vi "PH_VacuumControl.PC Set Trend Channel.vi"(0 "i ref in":refnum<vi>, 2 "Trend Channel":u16, 5 "error IO":errorcluster) -> (14 "i ref out":refnum<vi>, 19 "error out":errorcluster)   [LabVIEW 2014, in "PH_VacuumControl.lvlib"]
doc: "This VI sets the Trend Channel to own attributes and the related GUI element."
uses:
  PH_VacuumControl.lvlib
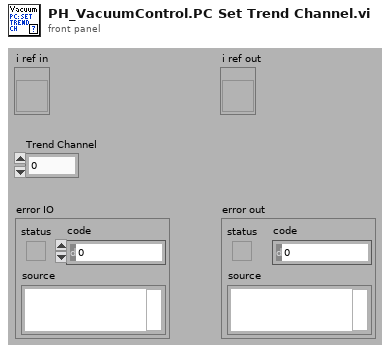
[diagram p1: front panel]
types:
  T1 = typedef "PH_VacuumControl.lvlib/PH_VacuumControl.i attribute.ctl" = cluster{"GUI Refs":cluster{"Exit":refnum<vi>, "Set Unit":refnum<vi>, "Device found":refnum<vi>, "Busy":refnum<vi>, "State":refnum<vi>, "Delete":refnum<vi>, "Channels":refnum<vi>, "Channel Name":refnum<vi>, "Trend":refnum<vi>, "Logarithmic":refnum<vi>, "Limit reached":refnum<vi>, "Channel Name 1 MT":refnum<vi>, "Channel Name 2 MT":refnum<vi>, "Trend MT":refnum<vi>, "Logarithmic MT":refnum<vi>, "Limit reached MT":refnum<vi>}, "Device found":bool, "Busy":bool, "Selected Unit":i32, "Channels [mbar]":T2, "Channel Names":cluster{"Channel 1":string, "Channel 2":string, "Channel 3":string, "Channel 4":string, "Channel 5":string, "Channel 6":string}, "Status":T3, "AGCxxx VISA Cluster":T4, "Instr Firmware Revision":string, "Service IDs Pressure":cluster{"Channel 1":i32, "Channel 2":i32, "Channel 3":i32, "Channel 4":i32, "Channel 5":i32, "Channel 6":i32}, "Service IDs Limits":cluster{"Channel 1":i32, "Channel 2":i32, "Channel 3":i32, "Channel 4":i32, "Channel 5":i32, "Channel 6":i32}, "Trend":cluster{"Start Point":timestamp, "Pressures [mbar] Channel 1":dbl[], "Pressures [mbar] Channel 2":dbl[], "Pressures [mbar] Channel 3":dbl[], "Pressures [mbar] Channel 4":dbl[], "Pressures [mbar] Channel 5":dbl[], "Pressures [mbar] Channel 6":dbl[], "Timebase [s]":i32[], "Trend Channel":u16, "Start Fit":dbl, "Trend Channel 1 MT":u16, "Trend Channel 2 MT":u16, "Start or continue Fit MT":dbl, "Continue or start Fit MT":dbl, "Datasets strored":i32, "Dataarray Size":i32}, "Running":bool}
  T2 = typedef "PH_VacuumControl.lvlib/PH_VacuumControl.Channels.ctl" = cluster{"Channel 1":dbl, "Channel 2":dbl, "Channel 3":dbl, "Channel 4":dbl, "Channel 5":dbl, "Channel 6":dbl, "Name Channel 1":string, "Name Channel 2":string, "Name Channel 3":string, "Name Channel 4":string, "Name Channel 5":string, "Name Channel 6":string, "Upper Limit":dbl, "Upper Limit 2":dbl, "Upper Limit 3":dbl, "Upper Limit 4":dbl, "Upper Limit 5":dbl, "Upper Limit 6":dbl}
  T3 = typedef "PH_StatusHandler.lvlib/PH_StatusHandler.Status.ctl" = i16
  T4 = typedef "AGCxxx - Driver.lvlib/AGCxxx VISA Control.ctl" = cluster{"VISA resource name":refnum<visa-resource-name>, "VISA Timeout Value (1000 ms)":u32, "Lock Timeout (1000 ms)":u32, "MAX Channel (6)":i32}
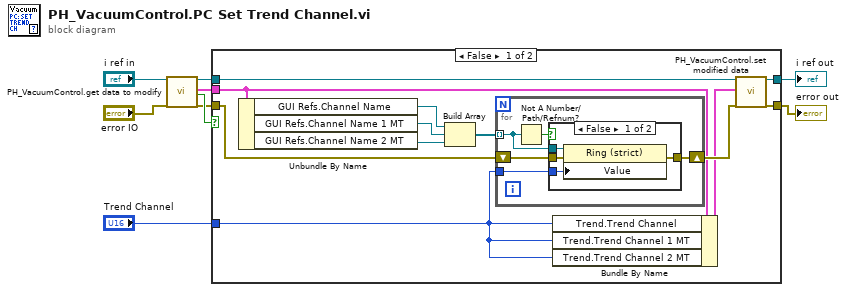
[diagram p0: block diagram]
diagram:
  n1 = call "PH_VacuumControl.get data to modify.vi"("i ref in"="i ref in", "error in (no error)"="error IO") -> ("i ref out"=w7:refnum<vi>, "i attribute"=w3:T1, "timed out"=w6:bool, "error out"=w4:errorcluster)  [unwired: 14 in]
  n2 = case shown="False" w6 {
    tunnel: w3 -> [w16 _]
    tunnel: w4 -> [w20 w32]
    tunnel: [w19 w32] -> w5
    tunnel: w7 -> [w18 w33]
    tunnel: [w17 w33] -> w8
    tunnel: "Trend Channel" -> [w14 _]
    frame False {
      n3 = Unbundle By Name(w16) -> ("GUI Refs.Channel Name"=w13:refnum<vi>, "GUI Refs.Channel Name 1 MT"=w11:refnum<vi>, "GUI Refs.Channel Name 2 MT"=w10:refnum<vi>)
      n4 = Build Array(w13, w11, w10) -> (w12:refnum<vi>[])
      n5 = for {
        tunnel: w14 -> [w23]
        tunnel: w12 -> [w22] mode=indexing
        shift-right: [w26] -> w21
        shift-left: w20 -> [w25]
        n6 = Not A Number/Path/Refnum?(number/path/refnum=w22) -> (NaN/Path/Refnum?=w24:bool)
        n7 = case shown="False" w24 {
          tunnel: [w30 w31] -> w26
          tunnel: w25 -> [w29 w31]
          tunnel: w22 -> [w28 _]
          tunnel: w23 -> [w27 _]
          frame False {
            n8 = property class="Ring (strict)"(reference=w28, error in=w29, "Value"=w27) -> (error out=w30:errorcluster)  [unwired: 1 out]
          }
          frame True {
          }
        }
      }
      n9 = Bundle By Name(cluster=w16, "Trend.Trend Channel"=w14, "Trend.Trend Channel 1 MT"=w14, "Trend.Trend Channel 2 MT"=w14) -> (w15:T1)
      n10 = call "PH_VacuumControl.set modified data.vi"("i ref in"=w18, "i attribute"=w15, "error in (no error)"=w21) -> ("i ref out"=w17:refnum<vi>, "error out"=w19:errorcluster)  [unwired: 15 in]
    }
    frame True {
    }
  }
  "i ref out" <- w8
  "error out" <- w5
